vi "MoveAxesAbsolute.vi"() -> ()   [LabVIEW 2015]
uses:
  <userlib>/Newport ESP301/Newport ESP301.lvlib
panel:
  in  "Position":dbl format="%#_13g"
  in  "Position":dbl format="%#_13g"
  in  "Position":dbl format="%#_13g"
  in  "Axis 3":bool
  in  "Axis 2":bool
  in  "Axis 1":bool
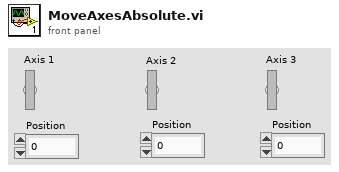
[diagram p1: front panel]
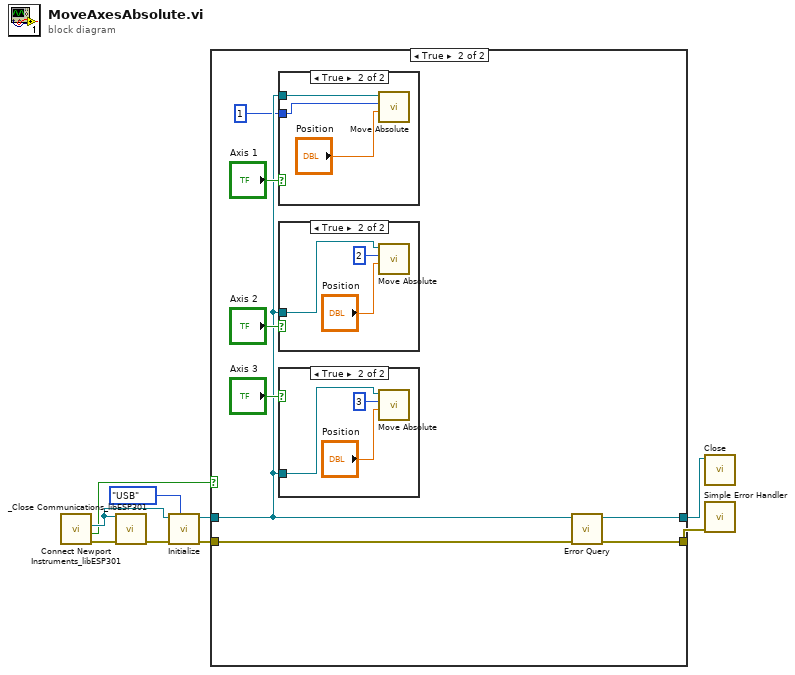
[diagram p0: block diagram]
diagram:
  n1 = call <userlib>:"Connect Newport Instruments_libESP301.vi"() -> ("error (duplicate)"=w7:errorcluster, "Connected"=w1:bool, "VISA resource name (duplicate)"=w6:refnum<visa-resource-name>)  [unwired: 7 in, 2 out]
  n2 = call <userlib>:"_Close Communications_libESP301.vi"("Instrument Channel"=w6, "error in (no error)"=w7) -> ("error out"=w9:errorcluster)  [unwired: 13 in]
  n3 = call <userlib>:"Initialize.vi"("VISA resource name"=w6, "error in (no error)"=w9, "Serial Link (USB)"=enum16{"RS232", "USB"}."USB" ("Serial Link (RS232)")) -> ("VISA resource name out"=w5:refnum<visa-resource-name>, "error out"=w4:errorcluster)  [unwired: 6 in]
  n4 = case shown="True" w1 {
    tunnel: w5 -> [w11 w13]
    tunnel: w4 -> [w10 w16]
    tunnel: [w11 w14] -> w3
    tunnel: [w10 w15] -> w2
    frame False {
    }
    frame True {
      n5 = case shown="True" "Axis 1" {
        tunnel: w13 -> [_ w28]
        tunnel: 1 -> [_ w26]
        frame False {
        }
        frame True {
          n6 = call <userlib>:"Move Absolute.vi"("Position (0 units)"="Position", "Axis (1)"=w26, "VISA resource name"=w28) -> ()  [unwired: 3 in, 2 out]
        }
      }
      n7 = case shown="True" "Axis 2" {
        tunnel: w13 -> [_ w24]
        frame False {
        }
        frame True {
          n8 = call <userlib>:"Move Absolute.vi"("Position (0 units)"="Position", "Axis (1)"=2, "VISA resource name"=w24) -> ()  [unwired: 3 in, 2 out]
        }
      }
      n9 = case shown="True" "Axis 3" {
        tunnel: w13 -> [_ w20]
        frame False {
        }
        frame True {
          n10 = call <userlib>:"Move Absolute.vi"("Position (0 units)"="Position", "Axis (1)"=3, "VISA resource name"=w20) -> ()  [unwired: 3 in, 2 out]
        }
      }
      n11 = call <userlib>:"Error Query.vi"("error in (no error)"=w16, "VISA resource name"=w13) -> ("error out"=w15:errorcluster, "VISA resource name out"=w14:refnum<visa-resource-name>)  [unwired: 2 in, 2 out]
    }
  }
  n12 = call <userlib>:"Close.vi"("VISA resource name"=w3) -> ()  [unwired: 10 in, 1 out]
  n13 = call <vilib>:"Simple Error Handler.vi"("error in (no error)"=w2) -> ()  [unwired: 1 in, 8 out]
